vi "DLL Download.vi"(2 "Overwrite":bool, 11 "Error In":errorcluster) -> (15 "Error Out":errorcluster)   [LabVIEW 2016]
doc: "This VI is used to download the correct PC Tools .NET DLLs that are required to use the Toolkit. Please run this VI prior to trying to use the toolkit"
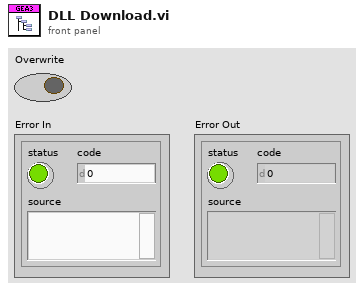
[diagram p1: front panel]
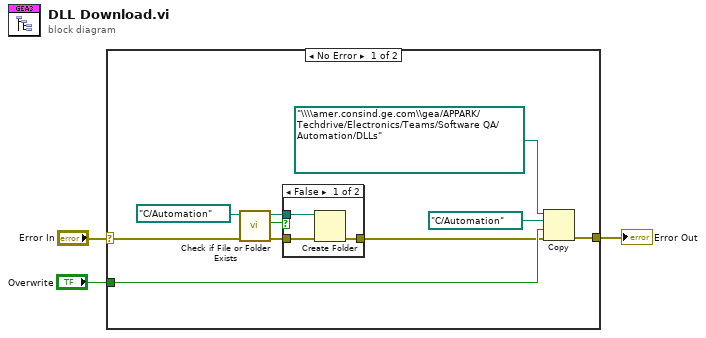
[diagram p0: block diagram]
diagram:
  n1 = case shown="No Error" "Error In" {
    selector: "Error In" -> [w11 w18]
    tunnel: [w4 w18] -> w3
    tunnel: "Overwrite" -> [w12 _]
    frame No Error {
      n2 = call <vilib>:"Check if File or Folder Exists.vi"("error in (no error)"=w11, "path"=path "C:/Automation" ("target path (use dialog)")) -> ("error out"=w9:errorcluster, "file or folder exists?"=w10:bool, "dup path"=w8:path)  [unwired: 7 in]
      n3 = case shown="False" w10 {
        tunnel: w9 -> [w16 w17]
        tunnel: w8 -> [w15 _]
        tunnel: [w14 w17] -> w7
        frame False {
          n4 = Create Folder(path (use dialog)=w15, error in=w16) -> (error out=w14:errorcluster)  [unwired: 1 in, 2 out]
        }
        frame True {
        }
      }
      n5 = Copy(8:w7, 9:w12, 10:path "C:/Automation" ("target path (use dialog)"), 11:path "\\\\amer.consind.ge.com\\gea/APPARK/Techdrive/Electronics/Teams/Software QA/Automation/DLLs" ("Product Source Path 2")) -> (0:w4:errorcluster)  [unwired: 1 in, 2 out]
    }
    frame Error {
    }
  }
  "Error Out" <- w3
